vi "SPD Get Results Test.vi"() -> ()   [LabVIEW 2018]
uses:
  <vilib>/Math Plots/3D Math Plots/3D Surface/3D Surface XCtrl/3D Surface.xctl
  SPD Stand/SubVIs/SPD.Params Selectors.ctl
  SPD Stand/typedefs/SPD.Stand Ctrl.ctl
  Instruments/SPD HID Interface/hidSPDLibForLabView/LibVIs/hidSPD Controls/hidSPD Device Session.ctl
  Instruments/SPD HID Interface/hidSPDLibForLabView/LibVIs/hidSPD Controls/hidSPD Controller.ctl
  Instruments/KC705 DevBoard/typedefs/DevB.Session.ctl
  Instruments/KeySight 53230A/typedefs/FreqC.Session.ctl
  Instruments/KeySight 8164B/KeySight 8164B LAN InstrLib/typedefs/KeySight 8164B control.ctl
  Instruments/LeCroy SDA830/typedefs/LeCroy.Session.ctl
  SPD Stand/typedefs/SPD.Events.ctl
  <vilib>/Utility/config.llb/Config Data RefNum.ctl
  SPD Stand/typedefs/SPD.Meas Result.ctl
  <vilib>/Math Plots/3D Math Plots/3D Surface/3D Surface Datatype/Public/Plot Helper (Vector).vi
  <vilib>/Math Plots/3D Math Plots/3D Surface/3D Surface Datatype/3D Surface Datatype.lvclass
  Instruments/SPD HID Interface/hidSPDLibForLabView/hidSPDLibForLabView.lvlib
  Instruments/KeySight 8164B/KeySight 8164B LAN InstrLib.lvlib
  <vilib>/Utility/config.llb/NI_LVConfig.lvlib
panel:
  in  "Result Tabs":enum32{"Graph", "Surface"}(tab)
  out "XY Graph":cluster{"HV_Bias":dbl[], dbl[]}[](graph)
  in  "ResultGraphSelector":enum32{"Item 0", "Item 1", "Radio Selection 3"}(radio) caption="Выбор Графика"
  in  "ParameterSelector":T1(radio) caption="Выбор Параметра"
  in  "ResultSurfaceSelector":enum32{"Item 0", "Item 1", "Radio Selection 3"}(radio) caption="Выбор Поверхности"
  out "Surface":refnum<class "3D Plot Datatype.lvclass">[](xcontrol) caption="Поверхность"
  in  "HV_bias_List":i32(listbox) caption="Смещение"
  in  "Stb_code_List":i32(listbox) caption="Код Строба"
  in  "Temperature_List":i32(listbox) caption="Температура"
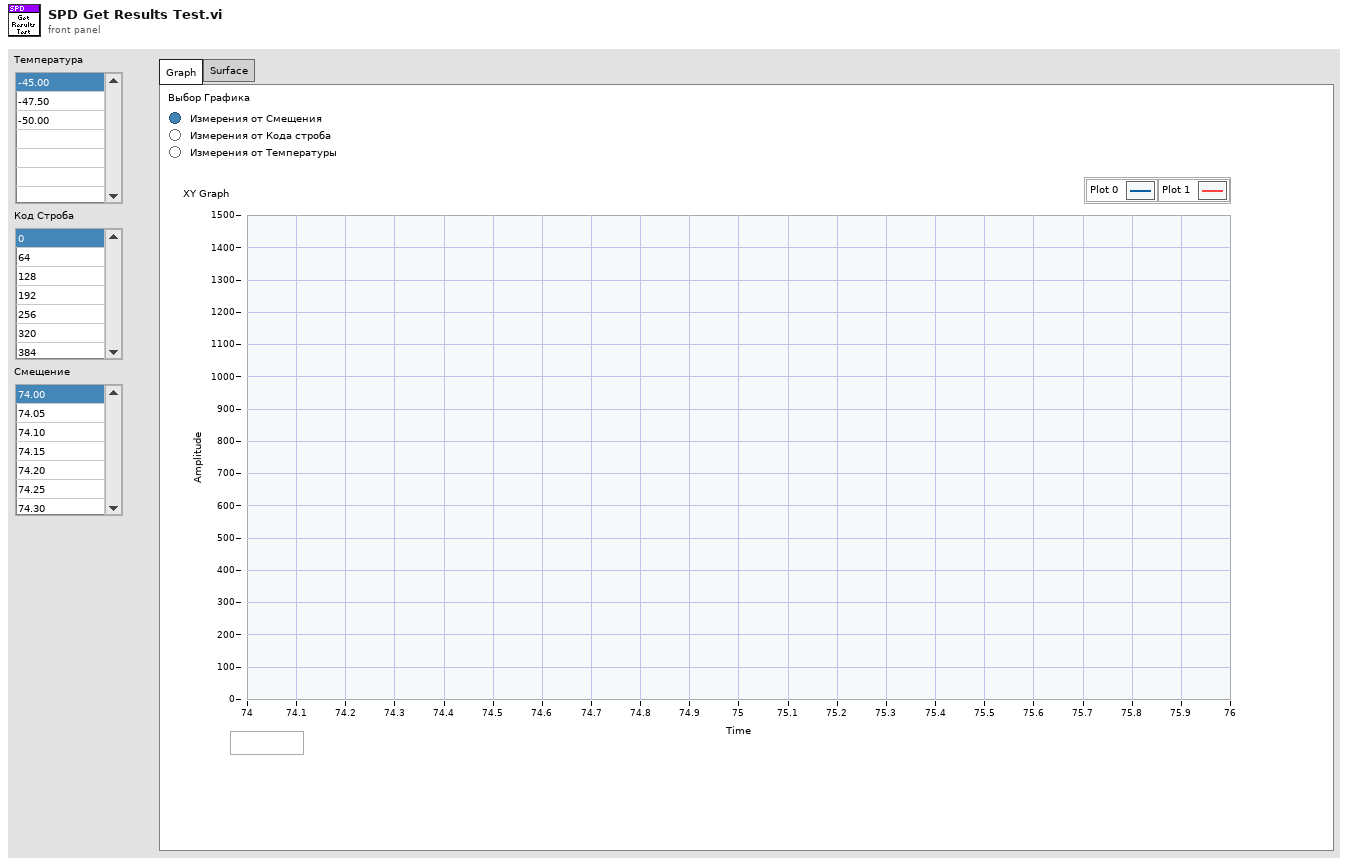
[diagram p1: front panel]
types:
  T1 = enum32{"Item 0", "Item 1", "Radio Selection 3", "Radio Selection 4"}
  T2 = typedef "SPD.Meas Result.ctl" = cluster{"HV_Bias":dbl[], "Stb_code":dbl[], "Temprature":dbl[], "Data":dbl[][][][]}
  T3 = typedef "SPD.Stand Ctrl.ctl" = cluster{"spdDeviceSession":T4, "DevBSession":T6, "FreqCSession":T7, "8164BSession":T8, "LeCroySession":T9, "Events":T10, "configFile":T11, "SPD.Result":T2}
  T4 = typedef "hidSPDLibForLabView.lvlib/hidSPD Device Session.ctl" = cluster{"spdRef":u64, "connected":bool, "spdName":string, "hidSPD.Controller":T5}
  T5 = typedef "hidSPDLibForLabView.lvlib/hidSPD Controller.ctl" = cluster{"TSet":sgl, "HV_bias":sgl, "DDS_stb_code":u16}
  T6 = typedef "DevB.Session.ctl" = cluster{"DevBRef":refnum<visa-resource-name>, "connected":bool}
  T7 = typedef "FreqC.Session.ctl" = cluster{"FreqCRef":refnum<visa-resource-name>, "timeout":dbl, "connected":bool}
  T8 = typedef "KeySight 8164B LAN InstrLib.lvlib/KeySight 8164B control.ctl" = cluster{"Connection ID":refnum<k5>, "Connected":bool, "Info":string, "Slots Info":string[]}
  T9 = typedef "LeCroy.Session.ctl" = cluster{"LeCroySession":refnum<visa-resource-name>, "connected":bool}
  T10 = typedef "SPD.Events.ctl" = cluster{"DCRTest":refnum<user-event>, "Stop":refnum<user-event>}
  T11 = typedef "NI_LVConfig.lvlib/Config Data RefNum.ctl" = refnum<k1>
  T12 = typedef "SPD.Params Selectors.ctl" = cluster{"HV_bias":i32, "Stb_code":i32, "Temperature":i32}
  T13 = typedef "SPD.Surface Plot.ctl" = cluster{"X":dbl[], "Y":dbl[], "Surface":dbl[][]}
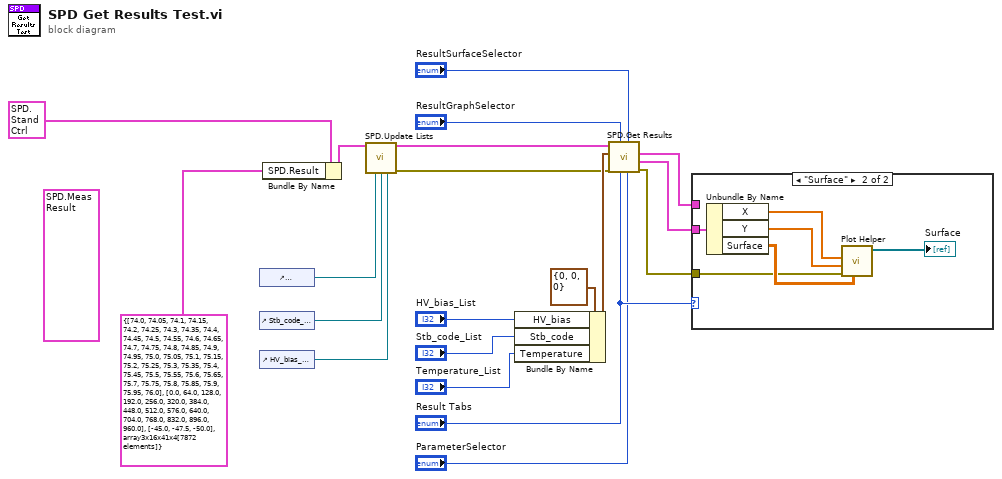
[diagram p0: block diagram]
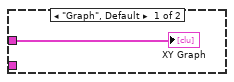
[diagram p2: hidden frame]
diagram:
  (unwired) T2 {"HV_Bias"=[74.5, 74.75, 75.0, 75.25, 75.5, 75.75, 76.0, 76.25, 76.5, 76.75, 77.0, 77.25, 77.5, 77.75, 78.0, 78.25, 78.5], "Stb_code"=[0.0, 5.0, 10.0, 15.0, 20.0], "Temprature"=[-45.0], "Data"=[[[[0.0, 0.0, nan, nan], [0.0057, 5.0, nan, nan], [0.0297, 46.0, nan, nan], [0.060000000000000005, 247.0, nan, nan], [0.08990000000000001, 484.0, nan, nan], [0.1436, 785.0, nan, nan], [0.25920000000000004, 1564.0, nan, nan], [0.49690000000000006, 3982.0, nan, nan], [1.0604, 10259.0, nan, nan], [1.7251, 24431.0, nan, nan], [1.9333000000000002, 49252.0, nan, nan], [1.2204000000000002, 76998.0, nan, nan], [0.677, 97628.0, nan, nan], [0.48530000000000006, 109379.0, nan, nan], [0.0, 0.0, nan, nan], [0.0984, 124142.0, nan, nan], [0.047400000000000005, 130084.0, nan, nan]], [[0.0021000000000000003, 1.0, nan, nan], [0.0082, 19.0, nan, nan], [0.022000000000000002, 94.0, nan, nan], [0.0478, 254.0, nan, nan], [0.08020000000000001, 485.0, nan, nan], [0.1194, 935.0, nan, nan], [0.25780000000000003, 1734.0, nan, nan], [0.5014000000000001, 4423.0, nan, nan], [1.0758, 10775.0, nan, nan], [1.8048000000000002, 25545.0, nan, nan], [1.5738, 52848.0, nan, nan], [1.1720000000000002, 77752.0, nan, nan], [0.7036, 97055.0, nan, nan], [-2.0323, 111539.0, nan, nan], [0.2886, 116447.0, nan, nan], [0.08750000000000001, 124989.0, nan, nan], [0.045500000000000006, 130639.0, nan, nan]], [[0.0029000000000000002, 1.0, nan, nan], [0.0097, 27.0, nan, nan], [0.024200000000000003, 92.0, nan, nan], [0.0279, 285.0, nan, nan], [0.0053, 490.0, nan, nan], [0.005, 866.0, nan, nan], [0.021, 1799.0, nan, nan], [0.0821, 4062.0, nan, nan], [0.2192, 10443.0, nan, nan], [0.5087, 24773.0, nan, nan], [0.5955, 49922.0, nan, nan], [0.7339000000000001, 74341.0, nan, nan], [0.4364, 95307.0, nan, nan], [0.44100000000000006, 107467.0, nan, nan], [0.15350000000000003, 118415.0, nan, nan], [0.0, 0.0, nan, nan], [0.10700000000000001, 128970.0, nan, nan]], [[0.0005, 0.0, nan, nan], [0.0021000000000000003, 17.0, nan, nan], [0.021500000000000002, 99.0, nan, nan], [0.0753, 277.0, nan, nan], [0.1121, 546.0, nan, nan], [0.1849, 757.0, nan, nan], [0.3164, 1719.0, nan, nan], [0.6038, 4330.0, nan, nan], [1.1717000000000002, 11344.0, nan, nan], [1.7389000000000001, 25337.0, nan, nan], [1.8706000000000003, 49183.0, nan, nan], [1.4923000000000002, 74499.0, nan, nan], [0.7411000000000001, 96655.0, nan, nan], [0.36060000000000003, 110408.0, nan, nan], [-9.5114, 119826.0, nan, nan], [0.14400000000000002, 123468.0, nan, nan], [0.07260000000000001, 129744.0, nan, nan]], [[0.0, 0.0, nan, nan], [0.0151, 17.0, nan, nan], [0.027600000000000003, 82.0, nan, nan], [0.06340000000000001, 222.0, nan, nan], [0.08720000000000001, 505.0, nan, nan], [0.135, 797.0, nan, nan], [0.2574, 1824.0, nan, nan], [0.5489, 4202.0, nan, nan], [1.1496000000000002, 10823.0, nan, nan], [1.8461, 24482.0, nan, nan], [1.6009000000000002, 50956.0, nan, nan], [1.5015, 74684.0, nan, nan], [0.7001000000000001, 97306.0, nan, nan], [0.26230000000000003, 111464.0, nan, nan], [-5.8264000000000005, 58264.0, nan, nan], [0.1272, 124191.0, nan, nan], [0.0492, 130439.0, nan, nan]]]]} ("SPD.Result")
  n1 = control-ref of="Temperature_List"() -> (w7:refnum<vi>)
  n2 = control-ref of="Stb_code_List"() -> (w6:refnum<vi>)
  n3 = control-ref of="HV_bias_List"() -> (w5:refnum<vi>)
  n4 = Bundle By Name(cluster=T3 {"spdDeviceSession"={"spdRef"=0, "connected"=FALSE, "spdName"="", "hidSPD.Controller"={"TSet"=0.0, "HV_bias"=0.0, "DDS_stb_code"=0}}, "DevBSession"={"DevBRef"="", "connected"=FALSE}, "FreqCSession"={"FreqCRef"="", "timeout"=0.0, "connected"=FALSE}, "8164BSession"={"Connection ID"=refnum, "Connected"=FALSE, "Info"="", "Slots Info"=[]}, "LeCroySession"={"LeCroySession"="", "connected"=FALSE}, "Events"={"DCRTest"=refnum, "Stop"=refnum}, "configFile"=refnum, "SPD.Result"={"HV_Bias"=[], "Stb_code"=[], "Temprature"=[], "Data"=[]}} ("SPD.Stand Ctrl in"), "SPD.Result"=T2 {"HV_Bias"=[74.0, 74.05, 74.1, 74.15, 74.2, 74.25, 74.3, 74.35, 74.4, 74.45, 74.5, 74.55, 74.6, 74.65, 74.7, 74.75, 74.8, 74.85, 74.9, 74.95, 75.0, 75.05, 75.1, 75.15, 75.2, 75.25, 75.3, 75.35, 75.4, 75.45, 75.5, 75.55, 75.6, 75.65, 75.7, 75.75, 75.8, 75.85, 75.9, 75.95, 76.0], "Stb_code"=[0.0, 64.0, 128.0, 192.0, 256.0, 320.0, 384.0, 448.0, 512.0, 576.0, 640.0, 704.0, 768.0, 832.0, 896.0, 960.0], "Temprature"=[-45.0, -47.5, -50.0], "Data"=array3x16x41x4[7872 elements]}) -> (w10:T3)
  n5 = call "SPD.Update Lists.vi"("SPD.Stand Ctrl in"=w10, "Temperature_List"=w7, "Stb_code_List"=w6, "HV_bias_List"=w5) -> ("SPD.Stand Ctrl out"=w9:T3, "Error Out"=w8:errorcluster)  [unwired: 10 in]
  n6 = Bundle By Name(cluster=T12 {"HV_bias"=0, "Stb_code"=0, "Temperature"=0} ("SPD.Parameter Selector"), "HV_bias"="HV_bias_List", "Stb_code"="Stb_code_List", "Temperature"="Temperature_List") -> (w18:T12)
  n7 = call "SPD.Get Results.vi"("ParameterSelector"="ParameterSelector", "SurfaceSelector"="ResultSurfaceSelector", "View Selector"="Result Tabs", "GraphSelector"="ResultGraphSelector", "Error In"=w8, "SPD.Parameter Selector"=w18, "SPD.Stand Ctrl in"=w9) -> ("Error Out"=w3:errorcluster, "SPD.Surface Plot"=w4:T13, "Graph Result"=w14:cluster{"HV_Bias":dbl[], dbl[]}[])  [unwired: 1 in, 1 out]
  n8 = case shown="\"Surface\"" "Result Tabs" {
    tunnel: w14 -> [w21 _]
    tunnel: w4 -> [_ w26]
    tunnel: w3 -> [_ w22]
    frame "Graph", Default {
      "XY Graph" <- w21
    }
    frame "Surface" {
      n9 = Unbundle By Name(w26) -> ("X"=w25:dbl[], "Y"=w24:dbl[], "Surface"=w23:dbl[][])
      n10 = call-poly <vilib>:"Plot Helper.vi"("z matrix"=w23, "error in (no error)"=w22, "y vector"=w24, "x vector"=w25) -> ("3D Plot lvclass Array out"=→"Surface":refnum<class "3D Plot Datatype.lvclass">[])  [unwired: 2 in, 5 out]
    }
  }
